vi "HTML2DBNew.vi"(8 "error in (no error)":errorcluster) -> (0 "error out":errorcluster)   [LabVIEW 2012]
uses:
  Global1.vi
  <vilib>/addons/database/Connection.llb/DB Tools Open Connec (Path).vi
  <vilib>/addons/database/NI_Database_API.lvlib
panel:
  in  "input cluster 2":T1
  out "filenames":string[](array[string])
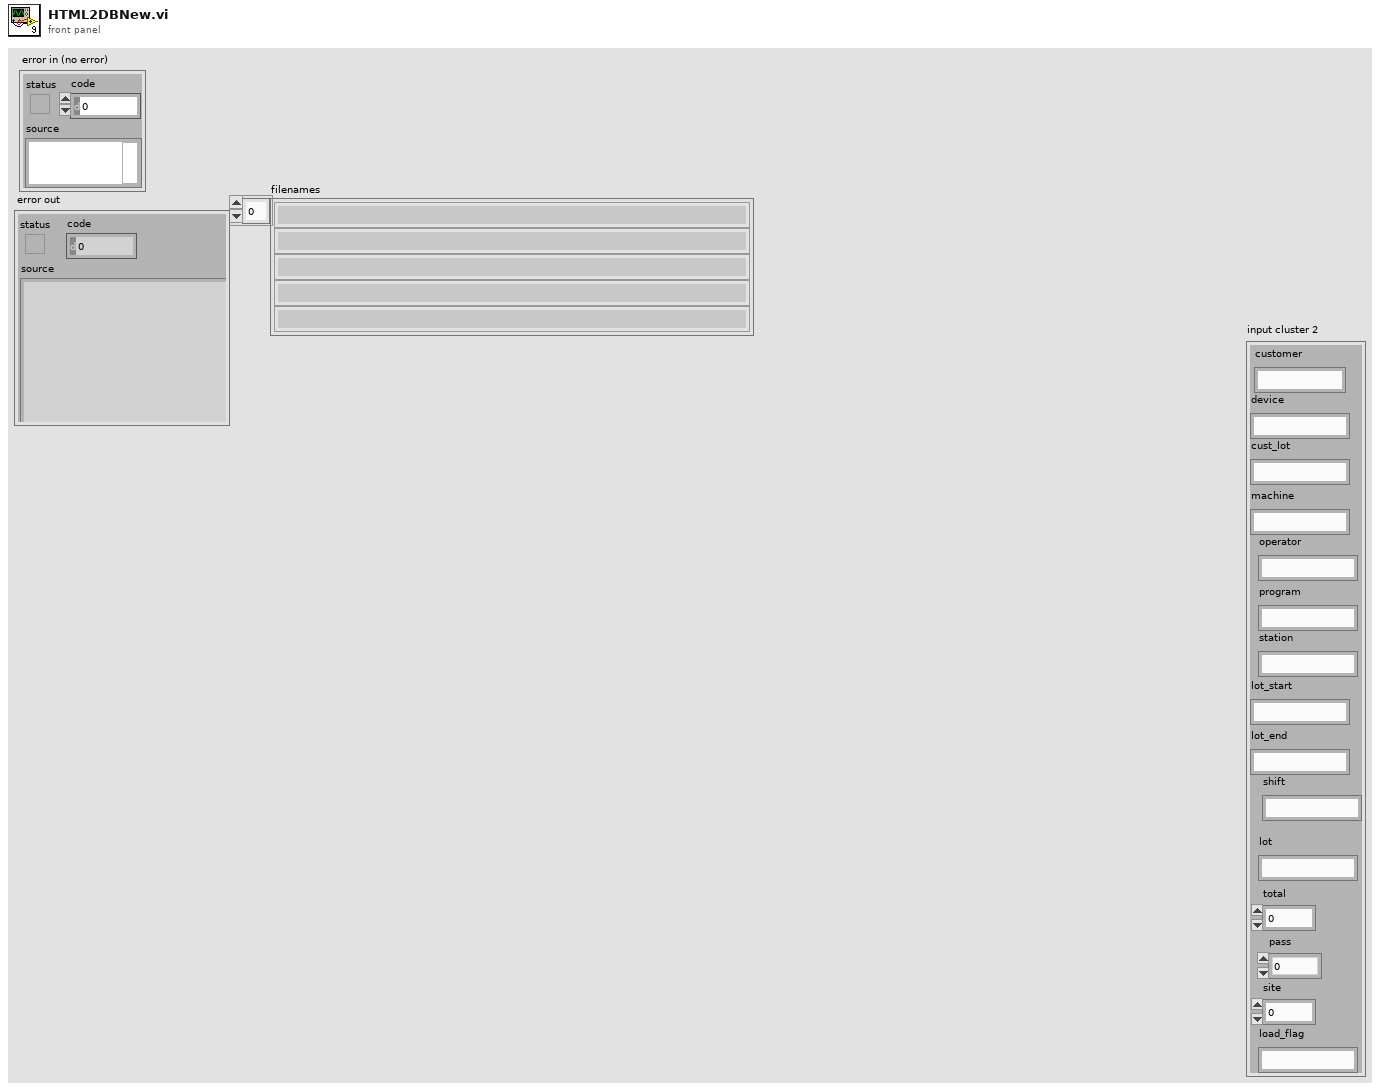
[diagram p1: front panel]
types:
  T1 = cluster{"customer":string, "device":string, "cust_lot":string, "machine":string, "operator":string, "program":string, "station":string, "lot_start":string, "lot_end":string, "shift":string, "lot":string, "total":dbl, "pass":dbl, "load_flag":string, "site":dbl}
  T2 = typedef "NI_Database_API.lvlib/Conn ObjectReference.ctl" = refnum<k1>
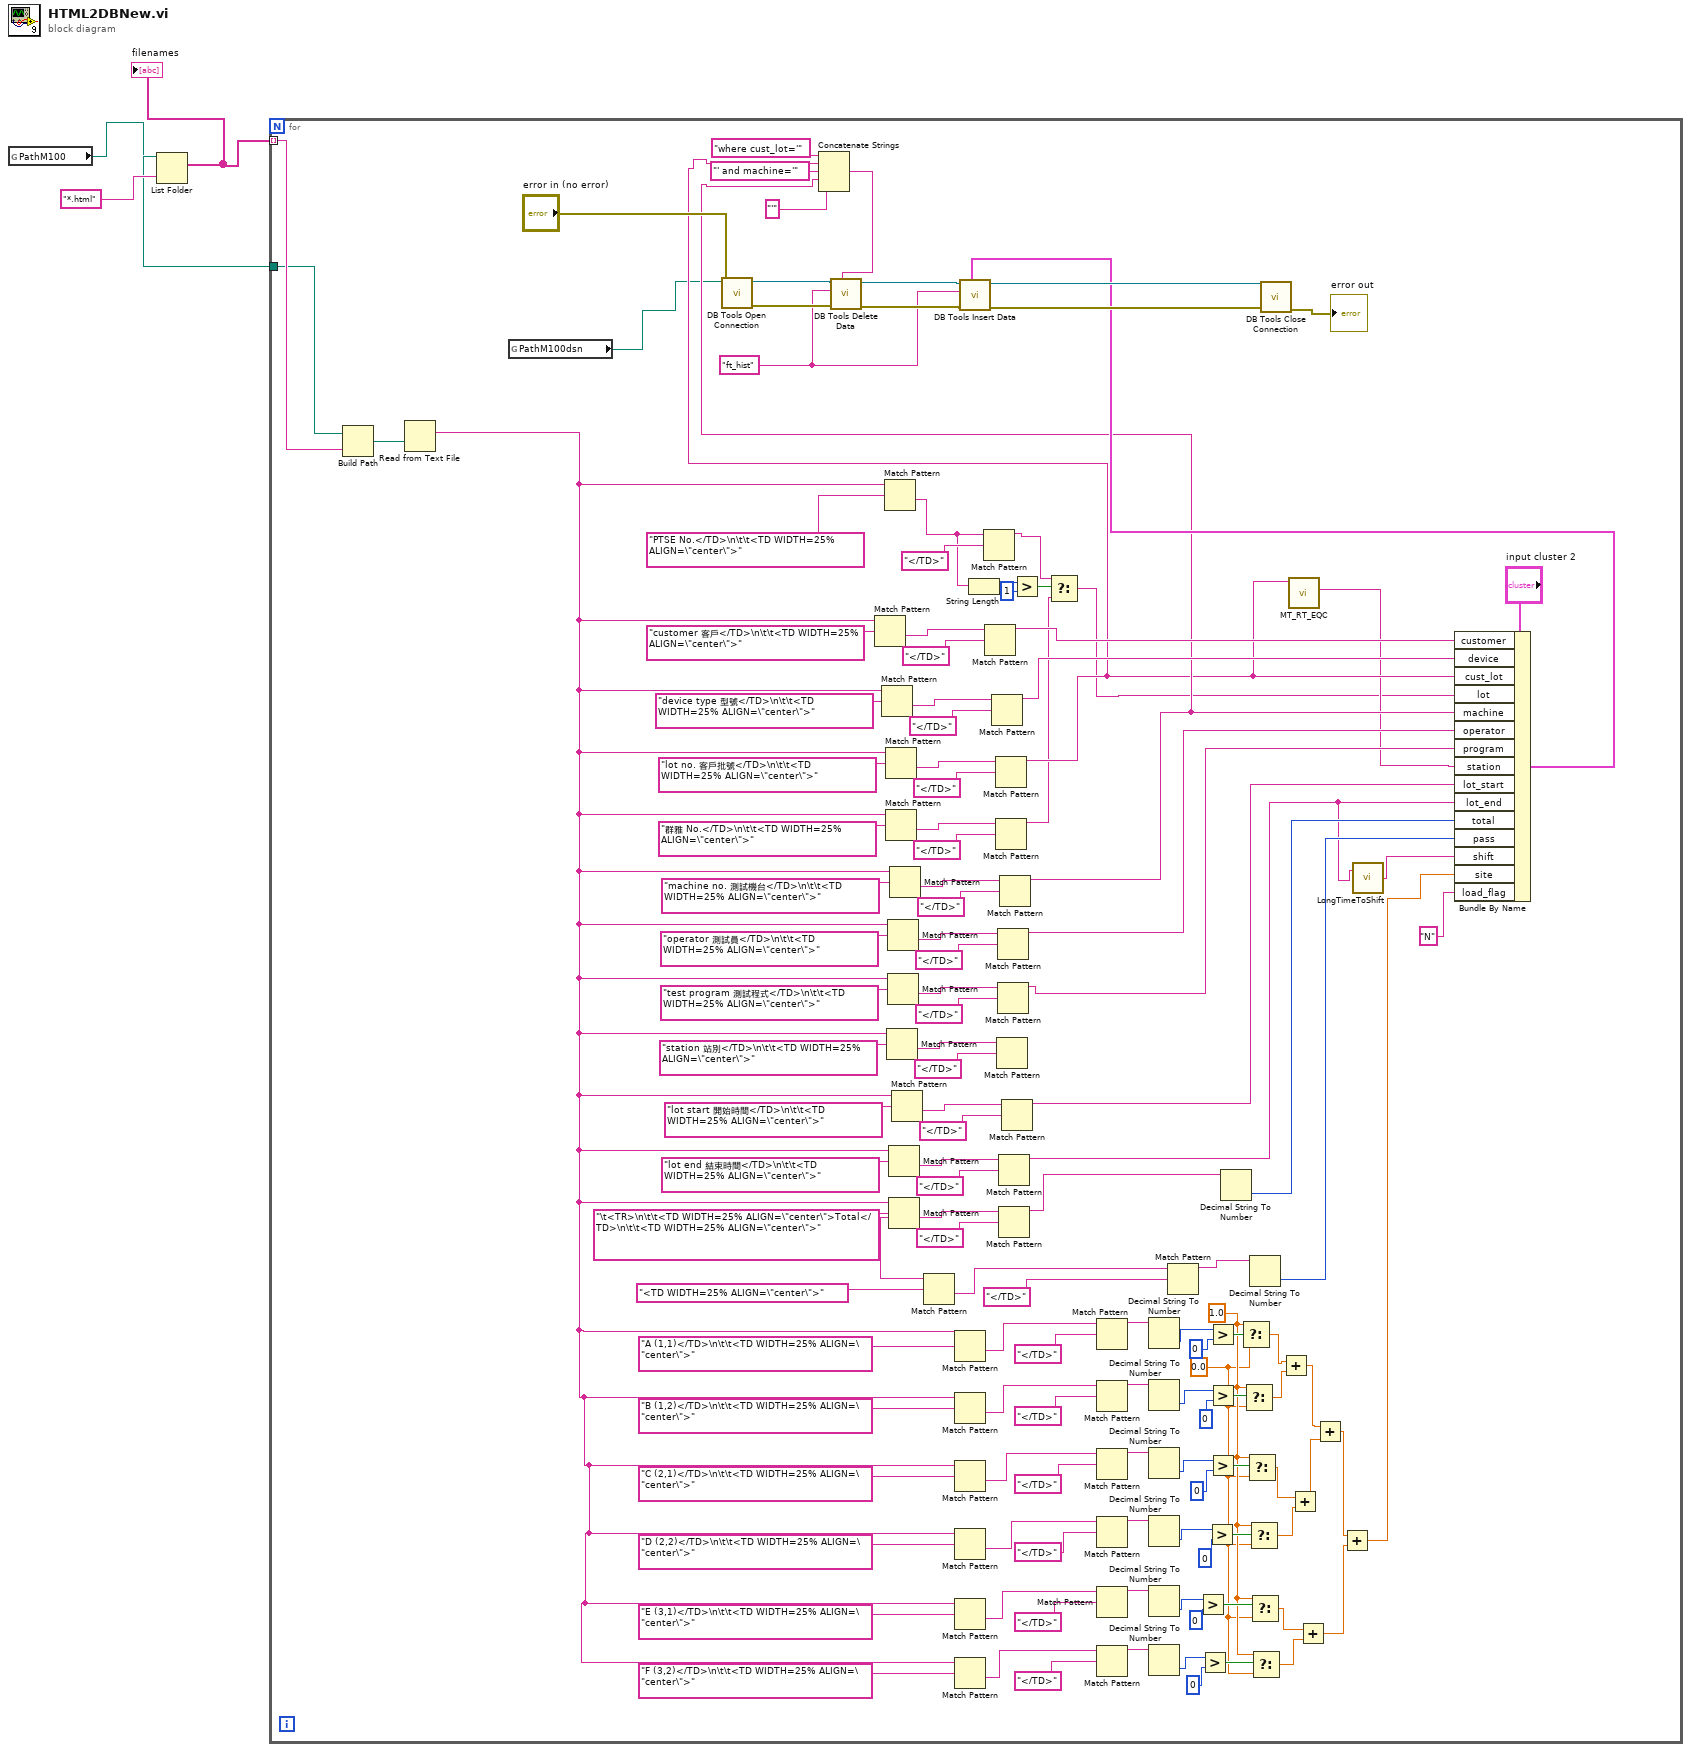
[diagram p0: block diagram]
diagram:
  n1 = global read "Global1.vi" "PathM100"() -> (w1:path)
  n2 = List Folder(path=w1, pattern="*.html") -> (path out=w2:path, filenames=w3:string[])  [unwired: 2 in, 2 out]
  "filenames" <- w3
  n3 = for {
    tunnel: w3 -> [w137] mode=indexing
    tunnel: w2 -> [w136]
    w36 = 0.0 ("f")
    w37 = 1.0 ("t")
    w80 = "ft_hist" ("table 2")
    n4 = Build Path(base path=w136, name or relative path=w137) -> (appended path=w138:path)
    n5 = Read from Text File(file (use dialog)=w138) -> (text=w5:string)  [unwired: 3 in, 3 out]
    n6 = global read "Global1.vi" "PathM100dsn"() -> (w15:path)
    n7 = call-poly <vilib>:"DB Tools Open Connection.vi"("error in (no error)"="error in (no error)", "connection information"=w15) -> ("error out"=w82:errorcluster, "connection reference"=w84:T2)  [unwired: 6 in]
    n8 = Match Pattern(string=w5, regular expression="customer 客戶</TD>\n\t\t<TD WIDTH=25% ALIGN=\"center\">") -> (after substring=w134:string)  [unwired: 1 in, 3 out]
    n9 = Match Pattern(string=w5, regular expression="device type 型號</TD>\n\t\t<TD WIDTH=25% ALIGN=\"center\">") -> (after substring=w131:string)  [unwired: 1 in, 3 out]
    n10 = Match Pattern(string=w5, regular expression="PTSE No.</TD>\n\t\t<TD WIDTH=25% ALIGN=\"center\">") -> (after substring=w12:string)  [unwired: 1 in, 3 out]
    n11 = Match Pattern(string=w5, regular expression="lot no. 客戶批號</TD>\n\t\t<TD WIDTH=25% ALIGN=\"center\">") -> (after substring=w128:string)  [unwired: 1 in, 3 out]
    n12 = Match Pattern(string=w5, regular expression="群雅 No.</TD>\n\t\t<TD WIDTH=25% ALIGN=\"center\">") -> (after substring=w125:string)  [unwired: 1 in, 3 out]
    n13 = Match Pattern(string=w5, regular expression="station 站別</TD>\n\t\t<TD WIDTH=25% ALIGN=\"center\">") -> (after substring=w113:string)  [unwired: 1 in, 3 out]
    n14 = Match Pattern(string=w5, regular expression="operator 測試員</TD>\n\t\t<TD WIDTH=25% ALIGN=\"center\">") -> (after substring=w119:string)  [unwired: 1 in, 3 out]
    n15 = Match Pattern(string=w5, regular expression="test program 測試程式</TD>\n\t\t<TD WIDTH=25% ALIGN=\"center\">") -> (after substring=w116:string)  [unwired: 1 in, 3 out]
    n16 = Match Pattern(string=w5, regular expression="lot end 結束時間</TD>\n\t\t<TD WIDTH=25% ALIGN=\"center\">") -> (after substring=w107:string)  [unwired: 1 in, 3 out]
    n17 = Match Pattern(string=w5, regular expression="\t<TR>\n\t\t<TD WIDTH=25% ALIGN=\"center\">Total</TD>\n\t\t<TD WIDTH=25% ALIGN=\"center\">") -> (after substring=w103:string)  [unwired: 1 in, 3 out]
    n18 = Match Pattern(string=w5, regular expression="machine no. 測試機台</TD>\n\t\t<TD WIDTH=25% ALIGN=\"center\">") -> (after substring=w122:string)  [unwired: 1 in, 3 out]
    n19 = Match Pattern(string=w5, regular expression="lot start 開始時間</TD>\n\t\t<TD WIDTH=25% ALIGN=\"center\">") -> (after substring=w110:string)  [unwired: 1 in, 3 out]
    n20 = Match Pattern(string=w103, regular expression="<TD WIDTH=25% ALIGN=\"center\">") -> (after substring=w100:string)  [unwired: 1 in, 3 out]
    n21 = Match Pattern(string=w5, regular expression="A (1,1)</TD>\n\t\t<TD WIDTH=25% ALIGN=\"center\">") -> (after substring=w72:string)  [unwired: 1 in, 3 out]
    n22 = Match Pattern(string=w5, regular expression="B (1,2)</TD>\n\t\t<TD WIDTH=25% ALIGN=\"center\">") -> (after substring=w67:string)  [unwired: 1 in, 3 out]
    n23 = Match Pattern(string=w5, regular expression="C (2,1)</TD>\n\t\t<TD WIDTH=25% ALIGN=\"center\">") -> (after substring=w63:string)  [unwired: 1 in, 3 out]
    n24 = Match Pattern(string=w5, regular expression="D (2,2)</TD>\n\t\t<TD WIDTH=25% ALIGN=\"center\">") -> (after substring=w59:string)  [unwired: 1 in, 3 out]
    n25 = Match Pattern(string=w5, regular expression="E (3,1)</TD>\n\t\t<TD WIDTH=25% ALIGN=\"center\">") -> (after substring=w55:string)  [unwired: 1 in, 3 out]
    n26 = Match Pattern(string=w5, regular expression="F (3,2)</TD>\n\t\t<TD WIDTH=25% ALIGN=\"center\">") -> (after substring=w51:string)  [unwired: 1 in, 3 out]
    n27 = String Length(string=w12) -> (length=w10:i32)
    n28 = Match Pattern(string=w12, regular expression="</TD>") -> (before substring=w8:string)  [unwired: 1 in, 3 out]
    n29 = Match Pattern(string=w134, regular expression="</TD>") -> (before substring=w97:string)  [unwired: 1 in, 3 out]
    n30 = Match Pattern(string=w131, regular expression="</TD>") -> (before substring=w96:string)  [unwired: 1 in, 3 out]
    n31 = Match Pattern(string=w128, regular expression="</TD>") -> (before substring=w17:string)  [unwired: 1 in, 3 out]
    n32 = Match Pattern(string=w125, regular expression="</TD>") -> (before substring=w7:string)  [unwired: 1 in, 3 out]
    n33 = Match Pattern(string=w113, regular expression="</TD>") -> ()  [unwired: 1 in, 4 out]
    n34 = Match Pattern(string=w119, regular expression="</TD>") -> (before substring=w95:string)  [unwired: 1 in, 3 out]
    n35 = Match Pattern(string=w116, regular expression="</TD>") -> (before substring=w94:string)  [unwired: 1 in, 3 out]
    n36 = Match Pattern(string=w107, regular expression="</TD>") -> (before substring=w90:string)  [unwired: 1 in, 3 out]
    n37 = Match Pattern(string=w103, regular expression="</TD>") -> (before substring=w99:string)  [unwired: 1 in, 3 out]
    n38 = Match Pattern(string=w122, regular expression="</TD>") -> (before substring=w77:string)  [unwired: 1 in, 3 out]
    n39 = Concatenate Strings("where cust_lot='" ("string"), w17, "' and machine='" ("string"), w77, "'" ("string")) -> (w75:string)
    n40 = call <vilib>:"DB Tools Delete Data.vi"("condition"=w75, "error in (no error)"=w82, "table"=w80, "connection reference"=w84) -> ("error out"=w81:errorcluster, "connection reference out"=w83:T2)  [unwired: 6 in]
    n41 = Match Pattern(string=w110, regular expression="</TD>") -> (before substring=w93:string)  [unwired: 1 in, 3 out]
    n42 = Greater?(x=w10, y=1) -> (0:w11:bool)
    n43 = Select(t=w8, s=w11, f=w7) -> (s? t:f=w6:string)
    n44 = Match Pattern(string=w72, regular expression="</TD>") -> (before substring=w70:string)  [unwired: 1 in, 3 out]
    n45 = Match Pattern(string=w67, regular expression="</TD>") -> (before substring=w66:string)  [unwired: 1 in, 3 out]
    n46 = Match Pattern(string=w63, regular expression="</TD>") -> (before substring=w62:string)  [unwired: 1 in, 3 out]
    n47 = Match Pattern(string=w59, regular expression="</TD>") -> (before substring=w58:string)  [unwired: 1 in, 3 out]
    n48 = Match Pattern(string=w55, regular expression="</TD>") -> (before substring=w54:string)  [unwired: 1 in, 3 out]
    n49 = Match Pattern(string=w51, regular expression="</TD>") -> (before substring=w50:string)  [unwired: 1 in, 3 out]
    n50 = Decimal String To Number(string=w70) -> (number=w21:i32)  [unwired: 2 in, 1 out]
    n51 = Decimal String To Number(string=w66) -> (number=w22:i32)  [unwired: 2 in, 1 out]
    n52 = Decimal String To Number(string=w62) -> (number=w23:i32)  [unwired: 2 in, 1 out]
    n53 = Decimal String To Number(string=w58) -> (number=w24:i32)  [unwired: 2 in, 1 out]
    n54 = Decimal String To Number(string=w54) -> (number=w25:i32)  [unwired: 2 in, 1 out]
    n55 = Decimal String To Number(string=w50) -> (number=w20:i32)  [unwired: 2 in, 1 out]
    n56 = Match Pattern(string=w100, regular expression="</TD>") -> (before substring=w71:string)  [unwired: 1 in, 3 out]
    n57 = Greater?(x=w25, y=0) -> (0:w39:bool)
    n58 = Greater?(x=w20, y=0) -> (0:w38:bool)
    n59 = Greater?(x=w24, y=0) -> (0:w40:bool)
    n60 = Greater?(x=w21, y=0) -> (0:w43:bool)
    n61 = Greater?(x=w22, y=0) -> (0:w42:bool)
    n62 = Greater?(x=w23, y=0) -> (0:w41:bool)
    n63 = Decimal String To Number(string=w99) -> (number=w92:i32)  [unwired: 2 in, 1 out]
    n64 = Select(t=w37, s=w43, f=w36) -> (s? t:f=w34:dbl)
    n65 = Select(t=w37, s=w42, f=w36) -> (s? t:f=w35:dbl)
    n66 = Select(t=w37, s=w41, f=w36) -> (s? t:f=w33:dbl)
    n67 = Select(t=w37, s=w40, f=w36) -> (s? t:f=w32:dbl)
    n68 = Decimal String To Number(string=w71) -> (number=w91:i32)  [unwired: 2 in, 1 out]
    n69 = Select(t=w37, s=w39, f=w36) -> (s? t:f=w31:dbl)
    n70 = Select(t=w37, s=w38, f=w36) -> (s? t:f=w30:dbl)
    n71 = Add(x=w34, y=w35) -> (x+y=w28:dbl)
    n72 = call "MT_RT_EQC.vi"("input string"=w17) -> ("Station"=w16:string)  [unwired: 6 in, 4 out]
    n73 = Add(x=w33, y=w32) -> (x+y=w29:dbl)
    n74 = Add(x=w31, y=w30) -> (x+y=w27:dbl)
    n75 = Add(x=w28, y=w29) -> (x+y=w26:dbl)
    n76 = Add(x=w26, y=w27) -> (x+y=w18:dbl)
    n77 = call "LongTimeToShift.vi"("input string"=w90) -> ("s? t:f"=w89:string)  [unwired: 1 in]
    n78 = Bundle By Name(cluster="input cluster 2", "customer"=w97, "device"=w96, "cust_lot"=w17, "lot"=w6, "machine"=w77, "operator"=w95, "program"=w94, "station"=w16, "lot_start"=w93, "lot_end"=w90, "total"=w92, "pass"=w91, "shift"=w89, "site"=w18, "load_flag"="N") -> (w86:T1)
    n79 = call <vilib>:"DB Tools Insert Data.vi"("data"=w86, "error in (no error)"=w81, "table"=w80, "connection reference"=w83) -> ("error out"=w87:errorcluster, "connection reference out"=w88:T2)  [unwired: 6 in]
    n80 = call <vilib>:"DB Tools Close Connection.vi"("error in (no error)"=w87, "connection reference"=w88) -> ("error out"=→"error out":errorcluster)  [unwired: 5 in]
  }
